vi "Motor control v0.5.vi"() -> ()   [LabVIEW 2016]
uses:
  C:/Users/Administrator/Downloads/LabVIEW/Kinesis/DLL Libraries/Thorlabs.MotionControl.Controls.dll
  DLL Libraries/Thorlabs.MotionControl.Controls.dll
  C:/Users/Administrator/Downloads/LabVIEW/Kinesis/DLL Libraries/Thorlabs.MotionControl.Benchtop.StepperMotorCLI.dll
  DLL Libraries/Thorlabs.MotionControl.Benchtop.StepperMotorCLI.dll
  C:/Users/Administrator/Downloads/LabVIEW/Kinesis/DLL Libraries/Thorlabs.MotionControl.GenericMotorCLI.dll
  DLL Libraries/Thorlabs.MotionControl.GenericMotorCLI.dll
panel:
  in  "Path":path=path "C:/users/rlp38/09Apr2009LTtesting/test2.txt"
  in  "Tab Control":enum32{"Main", "Other Parameters"}(tab)
  in  "stop":bool
  out "Elapsed Time":dbl caption="Elapsed Time (s)"
  in  "Units":u16(ring) items=["Seconds", "Minutes", "Hours"]
  in  "Time Offset":dbl caption="Set Start Time (s)"
  in  "Reset":bool
  in  "Auto Reset":bool
  out "Stage position vs time":cluster{"Y":dbl[], "Y":dbl[]}[](graph)
  in  "SerialNumber":string="40878702"
  in  "BenchtopStepperControl":refnum<k24>(container)
  out "error out":errorcluster
  in  "error in (no error)":errorcluster
  # "Time"
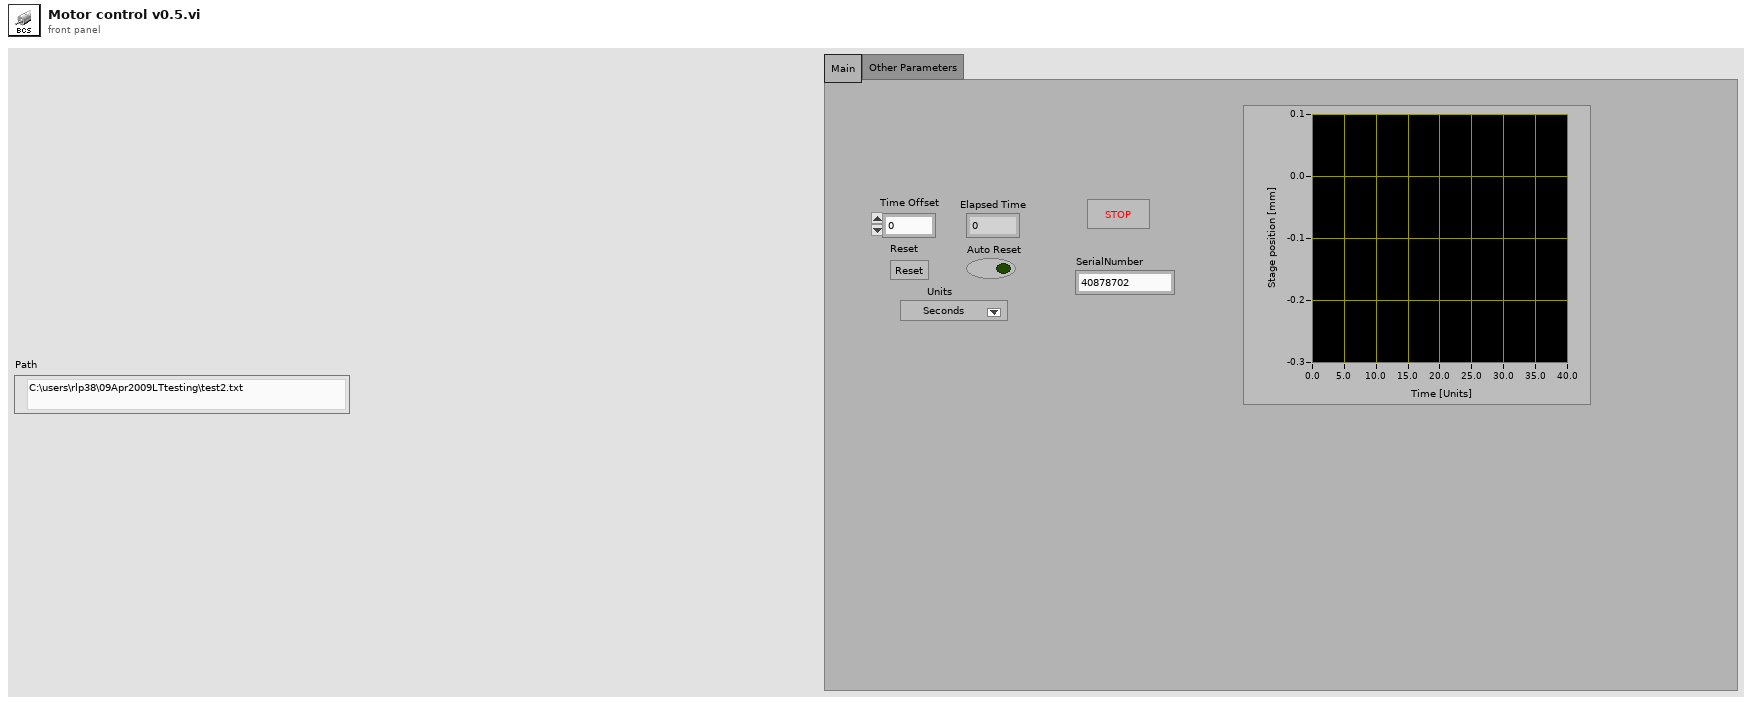
[diagram p1: front panel]
types:
  T1 = enum16{"open", "replace", "create", "open or create", "replace or create", "replace or create with confirmation"}
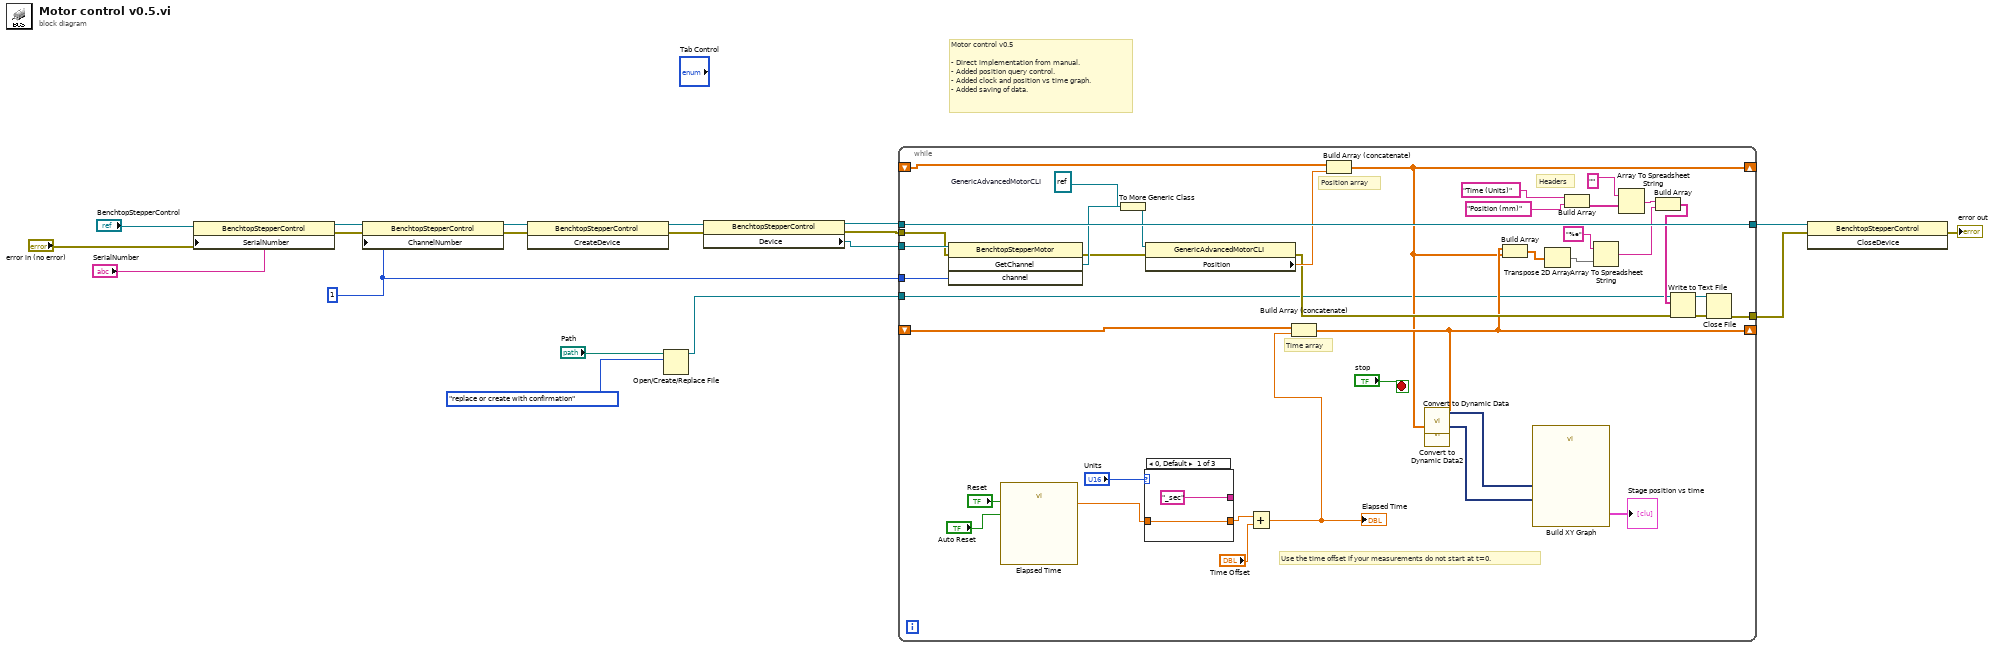
[diagram p0: block diagram]
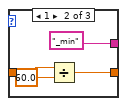
[diagram p2: hidden frame]
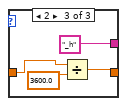
[diagram p3: hidden frame]
diagram:
  w7 = 1 ("ChannelNumber")
  # "Motor control v0.5\n\n- Direct implementation from manual.\n- Added position query control.\n- Added clock and position vs time graph.\n- Added saving of data."
  n1 = property class="BenchtopStepperControl"(reference="BenchtopStepperControl", error in="error in (no error)", "SerialNumber"="SerialNumber") -> (reference out=w11:refnum<k24>, error out=w10:errorcluster)
  n2 = property class="BenchtopStepperControl"(reference=w11, error in=w10, "ChannelNumber"=w7) -> (reference out=w9:refnum<k24>, error out=w8:errorcluster)
  n3 = invoke class="BenchtopStepperControl" method="CreateDevice"(reference=w9, error in=w8) -> (reference out=w15:refnum<k24>, error out=w12:errorcluster)  [unwired: 1 in, 1 out]
  n4 = Open/Create/Replace File(file path (use dialog)="Path", operation (0:open)=T1."replace or create with confirmation") -> (refnum out=w2:refnum<file>)  [unwired: 4 in, 2 out]
  n5 = property class="BenchtopStepperControl"(reference=w15, error in=w12) -> (reference out=w14:refnum<k24>, error out=w6:errorcluster, "Device"=w13:refnum<k24>)
  n6 = while {
    tunnel: w14 -> [w57]
    tunnel: [w57] -> w16
    tunnel: w13 -> [w56]
    tunnel: w7 -> [w55]
    shift-right: [w31] -> _
    shift-left: _ -> [w52]
    shift-right: [w30] -> _
    shift-left: _ -> [w50]
    tunnel: w6 -> [w39]
    tunnel: [w22] -> w4
    tunnel: w2 -> [w24]
    stop <- "stop" stop-if-true
    w20 = refnum<k24> refnum  # GenericAdvancedMotorCLI
    # "Headers"
    # "Use the time offset if your measurements do not start at t=0."
    # "Position array"
    # "Time array"
    n7 = invoke class="BenchtopStepperMotor" method="GetChannel"(reference=w56, error in=w39, "channel"=w55) -> (error out=w40:errorcluster, "GetChannel"=w54:refnum<k24>)  [unwired: 1 in, 2 out]
    n8 = call "Elapsed Time"("Reset"="Reset", "Auto Reset"="Auto Reset") -> ("Elapsed Time (s)"=w48:dbl)  [unwired: 10 in, 7 out]
    n9 = To More Generic Class(target class=w20, reference=w54) -> (generic class reference=w53:refnum<k24>)
    n10 = case shown="0, Default" "Units" {
      tunnel: ["_sec" "_min" "_h"] -> _
      tunnel: [w59 w63 w66] -> w44
      tunnel: w48 -> [w59 w62 w67]
      frame 0, Default {
      }
      frame 1 {
        n11 = Divide(x=w62, y=60.0) -> (x/y=w63:dbl)
      }
      frame 2 {
        n12 = Divide(x=w67, y=3600.0) -> (x/y=w66:dbl)
      }
    }
    n13 = property class="GenericAdvancedMotorCLI"(reference=w53, error in=w40) -> (error out=w38:errorcluster, "Position"=w51:dbl)  [unwired: 1 out]
    n14 = Add(x=w44, y="Time Offset") -> (x+y=w25:dbl)
    "Elapsed Time" <- w25
    n15 = Build Array (concatenate)(w52, w25) -> (w31:dbl[])
    n16 = Build Array (concatenate)(w50, w51) -> (w30:dbl[])
    n17 = call "Convert to Dynamic Data"("Array"=w31) -> ("Dynamic Data Type"=w42:dynamicdata)  [unwired: 3 in]
    n18 = call "Convert to Dynamic Data2"("Array"=w30) -> ("Dynamic Data Type"=w41:dynamicdata)  [unwired: 3 in]
    n19 = Build Array(w31, w30) -> (w27:dbl[][])
    n20 = call "Build XY Graph"("Y Input"=w41, "X Input"=w42) -> ("XY Graph"=→"Stage position vs time":cluster{"X":dbl[], "Y":dbl[]}[])  [unwired: 8 in, 1 out]
    n21 = Transpose 2D Array(2D array=w27) -> (transposed array=w26:dbl[][])
    n22 = Build Array("Time (Units)" ("element"), "Position (mm)" ("VAR2 Name")) -> (w35:string[])
    n23 = Array To Spreadsheet String(array=w26, 3:"%e" ("format string")) -> (spreadsheet string=w29:string)  [unwired: 1 in]
    n24 = Array To Spreadsheet String(array=w35, 3:"" ("format string")) -> (spreadsheet string=w32:string)  [unwired: 1 in]
    n25 = Build Array(w32, w29) -> (w28:string[])
    n26 = Write to Text File(file (use dialog)=w24, text=w28, error in=w38) -> (refnum out=w21:refnum<file>, error out=w23:errorcluster)  [unwired: 1 in, 1 out]
    n27 = Close File(refnum=w21, error in=w23) -> (error out=w22:errorcluster)  [unwired: 1 out]
  }
  n28 = invoke class="BenchtopStepperControl" method="CloseDevice"(reference=w16, error in=w4) -> (error out=→"error out":errorcluster)  [unwired: 1 in, 2 out]
